vi "DataFinder_ListIndexedValues.vi"(8 "error in (no error)":errorcluster, 10 "property":T1={"object type"=0, "property name"="", "data type"=23} {"data type" items=["Unknown"=0, "String"=23, "I32"=3, "I64"=4, "DBL"=10, "Time stamp"=30]; "object type" items=["File", "Channel Group", "Channel"]}, 11 "DataFinder":T4) -> (3 "Value":string)   [LabVIEW 2023]
doc: "This VI provides a list of indexed values for the specified property."
uses:
  <vilib>/userdefined/High Color/DFDataFinder.ctl
  <vilib>/DataFinder/DataTypes/property.ctl
  <vilib>/DataFinder/DataTypes/object type.ctl
  <vilib>/DataFinder/DataTypes/data type.ctl
  <vilib>/Utility/error.llb/DialogType.ctl
  <vilib>/DataFinder/NI_DataFinder.lvlib
  <vilib>/userdefined/NI_DataFinder Controls.lvlib
panel:
  out "error text":string=" INSTRUCTIONS:\r\rNormal Use:  When using subVIs that incorporate the error in/error out (or error I/O) structure, place this handler where you want to inform the user of an error, typically at the end of the I/O data path, as the last action of the program.  If the error in error? is ERROR, the handler creates a message describing the error and its source.  If the type of dialog = 1 (default), the message is displayed to the user, who can only acknowedge it.  If the type = 2, the user can acknowledge the message or abort execution; aborting a program with active I/O is not recommended.  If the type = 0, no message is displayed; this is used to process the error programmatically, and the error out cluster elements are wired to individual terminals for that reason.  \r\rOther Use:\n\r\nlocal testing.  To test the error code of a subVI or function that does not have the error I/O structure, you can wire its error code and a source string to the local error code and error source inputs.  If error in error? indicates no error and error code is not equal to 0, the local code and source are substituted for the error in values, and error? is set TRUE (ERROR)."
  in  "Table Control":string[][](table) caption="Indexed Values (175)"
  in  "Cancel":bool
  in  "OK":bool
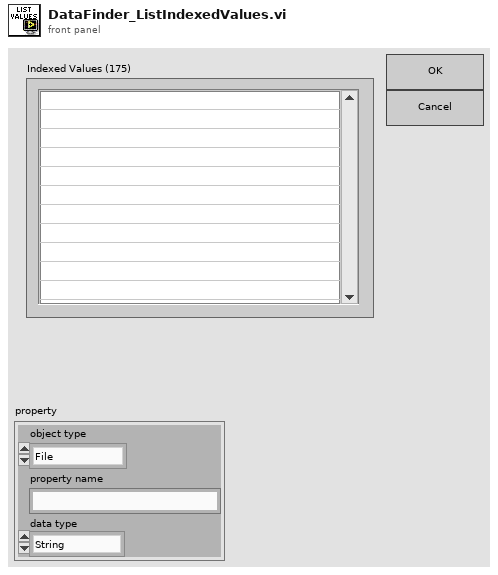
[diagram p1: front panel]
types:
  T1 = typedef "NI_DataFinder.lvlib/property.ctl" = cluster{"object type":T2, "property name":string, "data type":T3}
  T2 = typedef "NI_DataFinder.lvlib/object type.ctl" = u16
  T3 = typedef "NI_DataFinder.lvlib/data type.ctl" = u16
  T4 = typedef "NI_DataFinder Controls.lvlib/DFDataFinder.ctl" = refnum<k21>
  T5 = typedef "DialogType.ctl" = u16
  T6 = typedef "LVRowAndColumnTypeDef.ctl" = cluster{"Row":i32, "Column":i32}
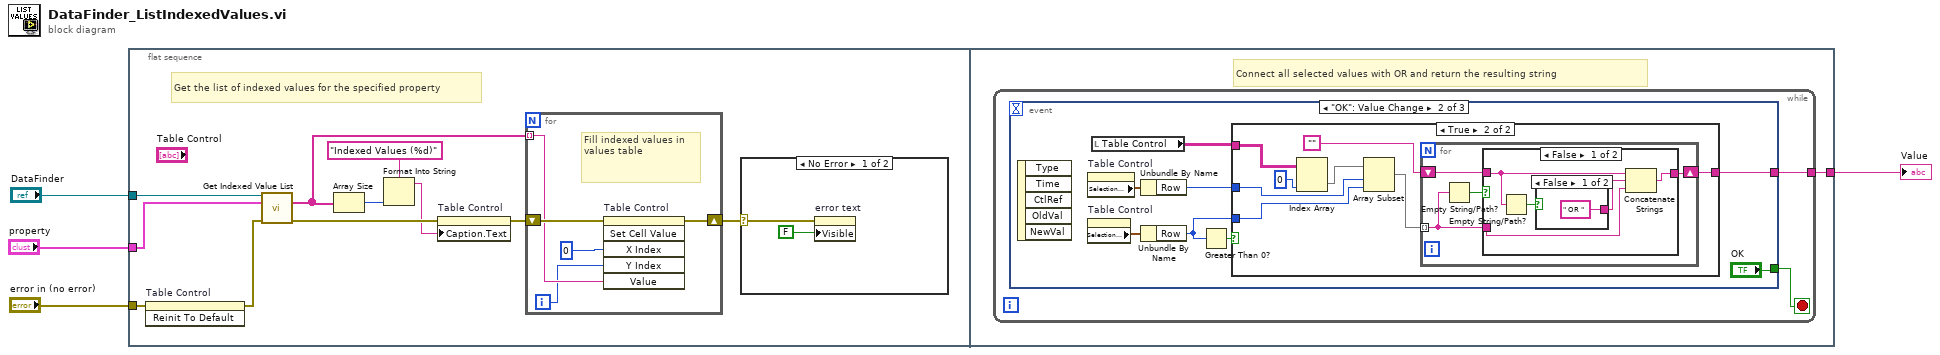
[diagram p0: block diagram]
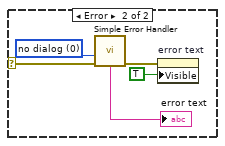
[diagram p2: hidden frame]
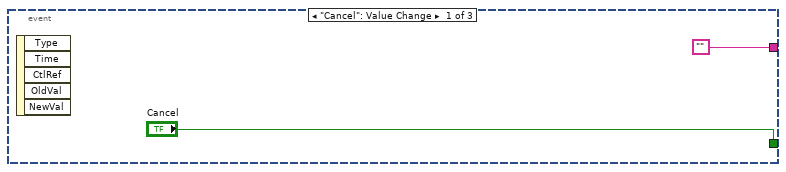
[diagram p3: hidden frame]
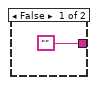
[diagram p4: hidden frame]
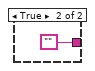
[diagram p5: hidden frame]
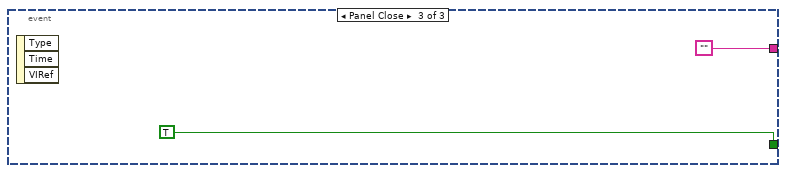
[diagram p7: hidden frame]
diagram:
  n1 = flat-sequence {
    tunnel: "DataFinder" -> [w15]
    tunnel: "property" -> [w8]
    tunnel: "error in (no error)" -> [w14]
    tunnel: [w28] -> w2
    frame #0 {
      # "Get the list of indexed values for the specified property"
      n2 = invoke on="Table Control" class="Tbl (strict)" method="Reinit To Default"(error in=w14) -> (error out=w13:errorcluster)  [unwired: 2 in, 2 out]
      n3 = call <vilib>:"Get Indexed Value List.vi"("DataFinder reference"=w15, "property"=w8, "error in (no error)"=w13) -> ("property values"=w11:string[], "error out"=w12:errorcluster)  [unwired: 8 in, 3 out]
      n4 = Array Size(array=w11) -> (size(s)=w7:i32)
      n5 = Format Into String(format string="Indexed Values (%d)" ("string"), w7) -> (resulting string=w5:string)  [unwired: 2 in, 1 out]
      n6 = property on="Table Control" class="Tbl (strict)"(error in=w12, "Caption.Text"=w5) -> (error out=w10:errorcluster)  [unwired: 1 in, 1 out]
      n7 = for {
        tunnel: w11 -> [w25] mode=indexing
        shift-right: [w26] -> w9
        shift-left: w10 -> [w27]
        i -> [w23]
        # "Fill indexed values in values table"
        n8 = invoke on="Table Control" class="Tbl (strict)" method="Set Cell Value"(error in=w27, "X Index"=u32 0, "Y Index"=w23, "Value"=w25) -> (error out=w26:errorcluster)  [unwired: 2 in, 5 out]
      }
      n9 = case shown="No Error" w9 {
        selector: w9 -> [w17 w22]
        frame No Error {
          n10 = property on="error text" class="Str"(error in=w17, "Visible"=FALSE) -> ()  [unwired: 1 in, 2 out]
        }
        frame Error {
          w21 = T5 0 items=["no dialog", "OK message", "continue or stop message", "OK message + warnings", "continue/stop + warnings"] ("type of dialog (OK msg:1)")
          n11 = call <vilib>:"Simple Error Handler.vi"("type of dialog (OK msg:1)"=w21, "error in (no error)"=w22) -> ("error out"=w18:errorcluster, "message"=→"error text":string)  [unwired: 6 out]
          n12 = property on="error text" class="Str"(error in=w18, "Visible"=TRUE) -> ()  [unwired: 1 in, 2 out]
        }
      }
    }
    frame #1 {
      # "Connect all selected values with OR and return the resulting string"
      n13 = while {
        tunnel: [w29] -> w28
        stop <- w30 stop-if-true
        n14 = event shown="[1] \"OK\": Value Change" {
          selector: _ -> [_ _ _]
          dyn-events: _ -> [_ _ _]
          timeout: _ -> [_ _ _]
          tunnel: ["Cancel" "OK" TRUE] -> w30
          tunnel: ["" w36 ""] -> w29
          event "Cancel": Value Change {
            n15 = event-data() -> ()  [unwired: 1 in, 5 out]
          }
          event "OK": Value Change {
            n16 = event-data() -> ()  [unwired: 1 in, 5 out]
            n17 = property on="Table Control" class="Tbl (strict)"() -> ("Selection Start"=w38:T6)  [unwired: 2 in, 2 out]
            n18 = property on="Table Control" class="Tbl (strict)"() -> ("Selection Size"=w37:T6)  [unwired: 2 in, 2 out]
            n19 = local read "Table Control"() -> (w33:string[][])
            n20 = Unbundle By Name(w38) -> ("Row"=w35:i32)
            n21 = Unbundle By Name(w37) -> ("Row"=w34:i32)
            n22 = Greater Than 0?(x=w34) -> (x > 0?=w39:bool)
            n23 = case shown="True" w39 {
              tunnel: ["" w47] -> w36
              tunnel: w33 -> [_ w46]
              tunnel: w35 -> [_ w44]
              tunnel: w34 -> [_ w43]
              frame False {
              }
              frame True {
                n24 = Index Array(array=w46, index (col)=0 ("disabled index (col)")) -> (element=w45:string[])  [unwired: 1 in]
                n25 = Array Subset(array=w45, index=w44, length=w43) -> (w49:string[])
                n26 = for {
                  tunnel: w49 -> [w51] mode=indexing
                  shift-right: [w52] -> w47
                  shift-left: "" -> [w53]
                  n27 = Empty String/Path?(string/path=w51) -> (empty?=w50:bool)
                  n28 = case shown="False" w50 {
                    tunnel: w53 -> [w54 w61]
                    tunnel: [w56 w61] -> w52
                    tunnel: w51 -> [w55 _]
                    frame False {
                      n29 = Empty String/Path?(string/path=w54) -> (empty?=w58:bool)
                      n30 = case shown="False" w58 {
                        tunnel: [" OR " ""] -> w57
                        frame False {
                        }
                        frame True {
                        }
                      }
                      n31 = Concatenate Strings(w54, w57, w55) -> (w56:string)
                    }
                    frame True {
                    }
                  }
                }
              }
            }
          }
          event Panel Close {
            n32 = event-data() -> ()  [unwired: 1 in, 3 out]
          }
        }
      }
    }
  }
  "Value" <- w2
